vi "calibrate pH.vi"(0 "index":i32, 1 "pH voltage":sgl format="%.2f", 2 "Temperature":sgl format="%.2f") -> (7 "Buffers":T1(array[cluster]) {"V/T" format="%.2f"; "Buffer" format="%.2f"})   [LabVIEW 2012]
uses:
  global scale array.vi
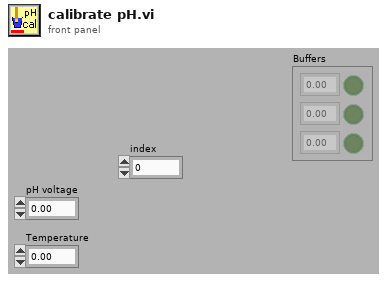
[diagram p1: front panel]
types:
  T1 = cluster{"Buffer":dbl, "Calibrated":bool, "V/T":dbl}[]
  T2 = enum16{"Volts", "Polynomial", "Correspondence Table", "pH", "Dissolved Oxygen"}
  T3 = typedef "calib array.ctl" = T4[]
  T4 = typedef "conversion.ctl" = cluster{"conversion matrix":sgl[][], "units":string, "name":string, "scale type":T5, "offset (volts)":dbl, "second channel":i8, "correspondence table":T6, "offset (physical units)":dbl, "pH scale":T7, "D.O.":T8}
  T5 = typedef "scale type.ctl" = enum16{"Volts", "Polynomial", "Correspondence Table", "pH", "Dissolved Oxygen", "Quadratic"}
  T6 = typedef "correspondence table.ctl" = cluster{"physical units":dbl, "volts":dbl}[]
  T7 = typedef "pH scale.ctl" = cluster{"Buffers":cluster{"Buffer":dbl, "Calibrated":bool, "V/T":dbl}[], "Temperature":dbl}
  T8 = typedef "DO scale.ctl" = cluster{"Temperature":dbl, "K":dbl, "barometric pressure":dbl}
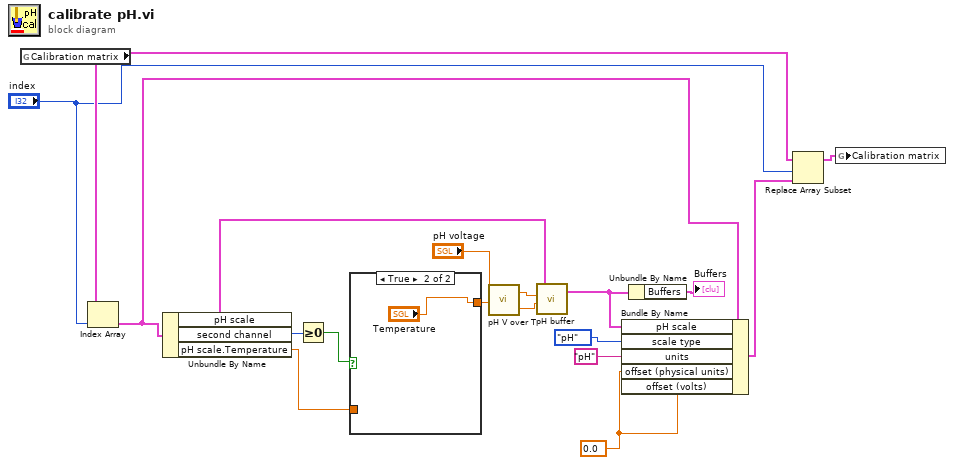
[diagram p0: block diagram]
diagram:
  w16 = 0.0 ("offset (physical units)")
  n1 = global read "global scale array.vi" "Calibration matrix"() -> (w8:T3)
  n2 = Index Array(array=w8, index="index") -> (element=w9:T4)
  n3 = Unbundle By Name(w9) -> ("pH scale"=w4:T7, "second channel"=w13:i8, "pH scale.Temperature"=w3:dbl)
  n4 = Greater Or Equal To 0?(x=w13) -> (x >= 0?=w14:bool)
  n5 = case shown="True" w14 {
    tunnel: [w19 "Temperature"] -> w15
    tunnel: w3 -> [w19 _]
    frame False {
    }
    frame True {
    }
  }
  n6 = call "pH V over T.vi"("Temperature"=w15, "Voltage"="pH voltage") -> ("Temperature out"=w11:dbl, "V/T"=w12:dbl)
  n7 = call "pH buffer.vi"("Temperature"=w11, "V/T"=w12, "pH scale in"=w4) -> ("pH scale out"=w2:T7)  [unwired: 1 in, 1 out]
  n8 = Bundle By Name(cluster=w9, "pH scale"=w2, "scale type"=T2."pH", "units"="pH", "offset (physical units)"=w16, "offset (volts)"=w16) -> (w5:T4)
  n9 = Unbundle By Name(w2) -> ("Buffers"=→"Buffers":T1)
  n10 = Replace Array Subset(array=w8, new element=w5, index="index") -> (w7:T3)
  n11 = global write "global scale array.vi" "Calibration matrix"(w7) -> ()
